vi "Init.vi"() -> (3 "Initialized DataBase":T1)   [LabVIEW 2019]
uses:
  #typedef_DataBase.ctl
  #typedef_SquareType.ctl
  #typedef_Color.ctl
  #typedef_Piece.ctl
  #typedef_PieceType.ctl
  #typedef_SquareLook.ctl
  #typedef_SpecialMoves.ctl
panel:
  out "?":u16[][](array[ring])
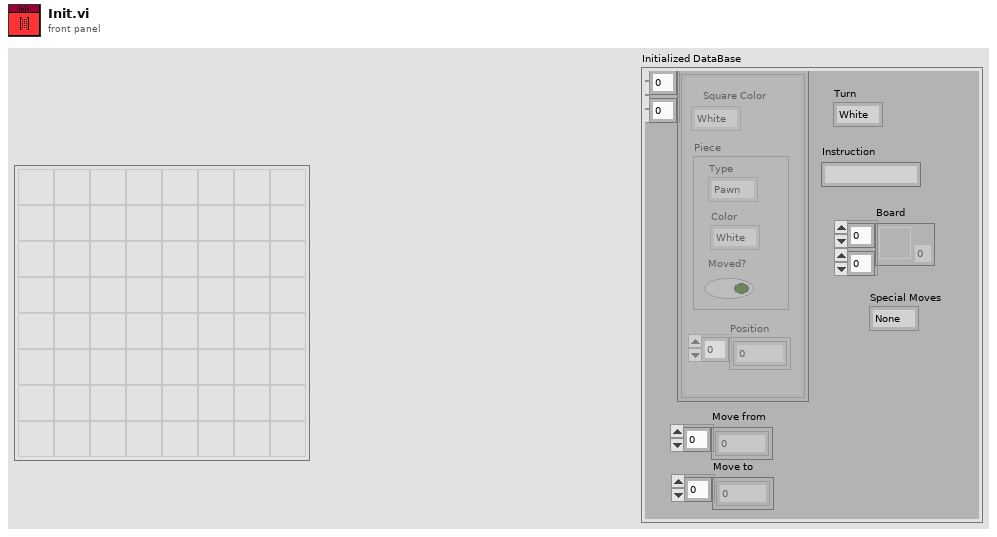
[diagram p1: front panel]
types:
  T1 = typedef "#typedef_DataBase.ctl" = cluster{"Squares type":T2[][], "Turn":T3, "Move from":i32[], "Move to":i32[], "Instruction":string, "Board":T6[][], "Special Moves":T7}
  T2 = typedef "#typedef_SquareType.ctl" = cluster{"Square Color":T3, "Position":i32[], "Piece":T4}
  T3 = typedef "#typedef_Color.ctl" = enum16{"White", "Black"}
  T4 = typedef "#typedef_Piece.ctl" = cluster{"Type":T5, "Color":T3, "Moved?":bool}
  T5 = typedef "#typedef_PieceType.ctl" = enum16{"None", "Pawn", "Knight", "Bishop", "Rook", "Queen", "King"}
  T6 = typedef "#typedef_SquareLook.ctl" = u16
  T7 = typedef "#typedef_SpecialMoves.ctl" = enum16{"None", "Last Square", "Beat in the Passage", "Short Castle", "Long Castle"}
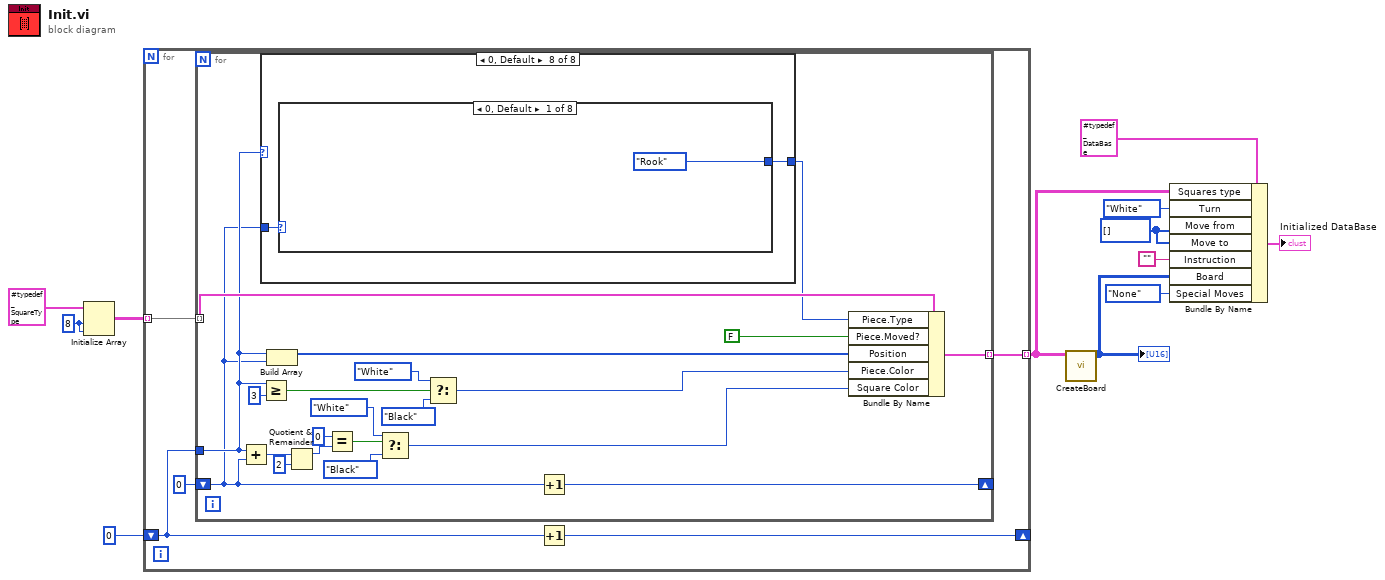
[diagram p0: block diagram]
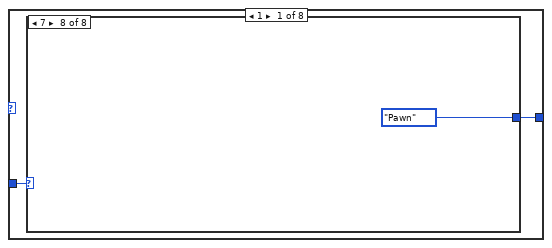
[diagram p2: hidden frame]
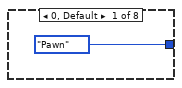
[diagram p3: hidden frame]
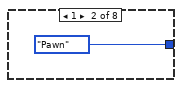
[diagram p4: hidden frame]
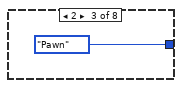
[diagram p5: hidden frame]
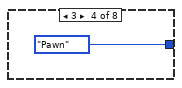
[diagram p6: hidden frame]
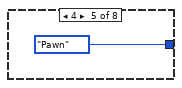
[diagram p7: hidden frame]
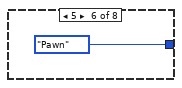
[diagram p8: hidden frame]
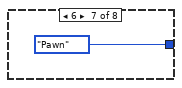
[diagram p9: hidden frame]
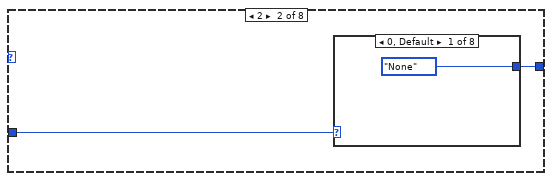
[diagram p10: hidden frame]
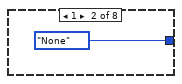
[diagram p11: hidden frame]
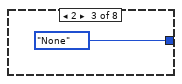
[diagram p12: hidden frame]
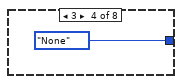
[diagram p13: hidden frame]
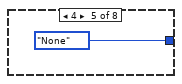
[diagram p14: hidden frame]
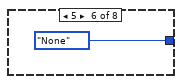
[diagram p15: hidden frame]
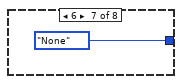
[diagram p16: hidden frame]
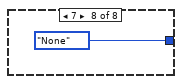
[diagram p17: hidden frame]
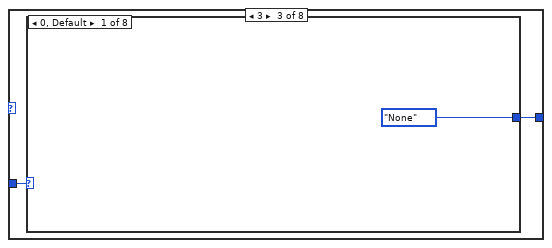
[diagram p18: hidden frame]
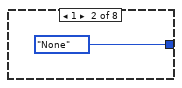
[diagram p19: hidden frame]
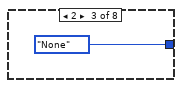
[diagram p20: hidden frame]
diagram:
  w5 = i32[] [] ("Move from")
  w9 = 8 ("dimension size")
  n1 = Initialize Array(T2 {"Square Color"=enum."White", "Position"=[], "Piece"={"Type"=enum."None", "Color"=enum."White", "Moved?"=FALSE}} ("Square Type"), w9, w9) -> (w11:T2[][])
  n2 = for {
    tunnel: w11 -> [w17] mode=indexing
    shift-right: [w16] -> _
    shift-left: 0 -> [w14]
    tunnel: [w13] -> w7 mode=indexing
    n3 = for {
      tunnel: w17 -> [w30] mode=indexing
      tunnel: w14 -> [w19]
      tunnel: [w20] -> w13 mode=indexing
      shift-right: [w38] -> _
      shift-left: 0 -> [w18]
      n4 = Add(x=w19, y=w18) -> (x+y=w37:i32)
      n5 = case shown="0, Default" w19 {
        tunnel: w18 -> [w40 w50 w60 w70 w80 w90 w100 w110]
        tunnel: [w39 w49 w59 w69 w79 w89 w99 w109] -> w21
        frame 1 {
          n6 = case shown="7" w40 {
            tunnel: [#typedef_PieceType."Pawn" ("Figure type") #typedef_PieceType."Pawn" ("Figure type") #typedef_PieceType."Pawn" ("Figure type") #typedef_PieceType."Pawn" ("Figure type") #typedef_PieceType."Pawn" ("Figure type") #typedef_PieceType."Pawn" ("Figure type") #typedef_PieceType."Pawn" ("Figure type") #typedef_PieceType."Pawn" ("Figure type")] -> w39
            frame 0, Default {
            }
            frame 1 {
            }
            frame 2 {
            }
            frame 3 {
            }
            frame 4 {
            }
            frame 5 {
            }
            frame 6 {
            }
            frame 7 {
            }
          }
        }
        frame 2 {
          n7 = case shown="0, Default" w50 {
            tunnel: [#typedef_PieceType."None" ("Figure type") #typedef_PieceType."None" ("Figure type") #typedef_PieceType."None" ("Figure type") #typedef_PieceType."None" ("Figure type") #typedef_PieceType."None" ("Figure type") #typedef_PieceType."None" ("Figure type") #typedef_PieceType."None" ("Figure type") #typedef_PieceType."None" ("Figure type")] -> w49
            frame 0, Default {
            }
            frame 1 {
            }
            frame 2 {
            }
            frame 3 {
            }
            frame 4 {
            }
            frame 5 {
            }
            frame 6 {
            }
            frame 7 {
            }
          }
        }
        frame 3 {
          n8 = case shown="0, Default" w60 {
            tunnel: [#typedef_PieceType."None" ("Figure type") #typedef_PieceType."None" ("Figure type") #typedef_PieceType."None" ("Figure type") #typedef_PieceType."None" ("Figure type") #typedef_PieceType."None" ("Figure type") #typedef_PieceType."None" ("Figure type") #typedef_PieceType."None" ("Figure type") #typedef_PieceType."None" ("Figure type")] -> w59
            frame 0, Default {
            }
            frame 1 {
            }
            frame 2 {
            }
            frame 3 {
            }
            frame 4 {
            }
            frame 5 {
            }
            frame 6 {
            }
            frame 7 {
            }
          }
        }
        frame 4 {
          n9 = case shown="4" w70 {
            tunnel: [#typedef_PieceType."None" ("Figure type") #typedef_PieceType."None" ("Figure type") #typedef_PieceType."None" ("Figure type") #typedef_PieceType."None" ("Figure type") #typedef_PieceType."None" ("Figure type") #typedef_PieceType."None" ("Figure type") #typedef_PieceType."None" ("Figure type") #typedef_PieceType."None" ("Figure type")] -> w69
            frame 0, Default {
            }
            frame 1 {
            }
            frame 2 {
            }
            frame 3 {
            }
            frame 4 {
            }
            frame 5 {
            }
            frame 6 {
            }
            frame 7 {
            }
          }
        }
        frame 5 {
          n10 = case shown="0, Default" w80 {
            tunnel: [#typedef_PieceType."None" ("Figure type") #typedef_PieceType."None" ("Figure type") #typedef_PieceType."None" ("Figure type") #typedef_PieceType."None" ("Figure type") #typedef_PieceType."None" ("Figure type") #typedef_PieceType."None" ("Figure type") #typedef_PieceType."None" ("Figure type") #typedef_PieceType."None" ("Figure type")] -> w79
            frame 0, Default {
            }
            frame 1 {
            }
            frame 2 {
            }
            frame 3 {
            }
            frame 4 {
            }
            frame 5 {
            }
            frame 6 {
            }
            frame 7 {
            }
          }
        }
        frame 6 {
          n11 = case shown="7" w90 {
            tunnel: [#typedef_PieceType."Pawn" ("Figure type") #typedef_PieceType."Pawn" ("Figure type") #typedef_PieceType."Pawn" ("Figure type") #typedef_PieceType."Pawn" ("Figure type") #typedef_PieceType."Pawn" ("Figure type") #typedef_PieceType."Pawn" ("Figure type") #typedef_PieceType."Pawn" ("Figure type") #typedef_PieceType."Pawn" ("Figure type")] -> w89
            frame 0, Default {
            }
            frame 1 {
            }
            frame 2 {
            }
            frame 3 {
            }
            frame 4 {
            }
            frame 5 {
            }
            frame 6 {
            }
            frame 7 {
            }
          }
        }
        frame 7 {
          n12 = case shown="6" w100 {
            tunnel: [#typedef_PieceType."Rook" ("Figure type") #typedef_PieceType."Knight" ("Figure type") #typedef_PieceType."Bishop" ("Figure type") #typedef_PieceType."Queen" ("Figure type") #typedef_PieceType."King" ("Figure type") #typedef_PieceType."Bishop" ("Figure type") #typedef_PieceType."Knight" ("Figure type") #typedef_PieceType."Rook" ("Figure type")] -> w99
            frame 0, Default {
            }
            frame 1 {
            }
            frame 2 {
            }
            frame 3 {
            }
            frame 4 {
            }
            frame 5 {
            }
            frame 6 {
            }
            frame 7 {
            }
          }
        }
        frame 0, Default {
          n13 = case shown="0, Default" w110 {
            tunnel: [#typedef_PieceType."Rook" ("Figure type") #typedef_PieceType."Knight" ("Figure type") #typedef_PieceType."Bishop" ("Figure type") #typedef_PieceType."Queen" ("Figure type") #typedef_PieceType."King" ("Figure type") #typedef_PieceType."Bishop" ("Figure type") #typedef_PieceType."Knight" ("Figure type") #typedef_PieceType."Rook" ("Figure type")] -> w109
            frame 0, Default {
            }
            frame 1 {
            }
            frame 2 {
            }
            frame 3 {
            }
            frame 4 {
            }
            frame 5 {
            }
            frame 6 {
            }
            frame 7 {
            }
          }
        }
      }
      n14 = Greater Or Equal?(x=w19, y=3) -> (x >= y?=w26:bool)
      n15 = Build Array(w19, w18) -> (w29:i32[])
      n16 = Quotient & Remainder(x=w37, y=2) -> (x-y*floor(x/y)=w35:i32)  [unwired: 1 out]
      n17 = Equal?(x=0, y=w35) -> (x = y?=w33:bool)
      n18 = Select(t=#typedef_Color."White" ("Color"), s=w33, f=#typedef_Color."Black") -> (s? t:f=w22:T3)
      n19 = Select(t=#typedef_Color."White" ("Color"), s=w26, f=#typedef_Color."Black") -> (s? t:f=w23:T3)
      n20 = Increment(x=w18) -> (x+1=w38:i32)
      n21 = Bundle By Name(cluster=w30, "Piece.Type"=w21, "Piece.Moved?"=FALSE, "Position"=w29, "Piece.Color"=w23, "Square Color"=w22) -> (w20:T2)
    }
    n22 = Increment(x=w14) -> (x+1=w16:i32)
  }
  n23 = call "CreateBoard.vi"("Squares type"=w7) -> ("Board"=w3:u16[][])  [unwired: 10 in]
  "?" <- w3
  n24 = Bundle By Name(cluster=T1 {"Squares type"=[], "Turn"=enum."White", "Move from"=[], "Move to"=[], "Instruction"="", "Board"=[], "Special Moves"=enum."None"} ("DataBase"), "Squares type"=w7, "Turn"=#typedef_Color."White", "Move from"=w5, "Move to"=w5, "Instruction"="", "Board"=w3, "Special Moves"=#typedef_SpecialMoves."None") -> (→"Initialized DataBase":T1)
